vi "RT-PC Main.vi"() -> ()   [LabVIEW 2021]
panel:
  in  "[ESC]":bool
  in  "my name":string="name"
  in  "clear messages":bool
  in  "send datagrams":bool
  in  "listening port":u16=50001
  in  "destination port":u16=50001
  in  "destination IP":string
  out "my primary IP address":string
  out "my available IP addresses":string[](array[string])
  out "number of addresses":i32
  out "received datagrams":string
  # "UDP ping"
  # "restart VI after changing\nlistening port number"
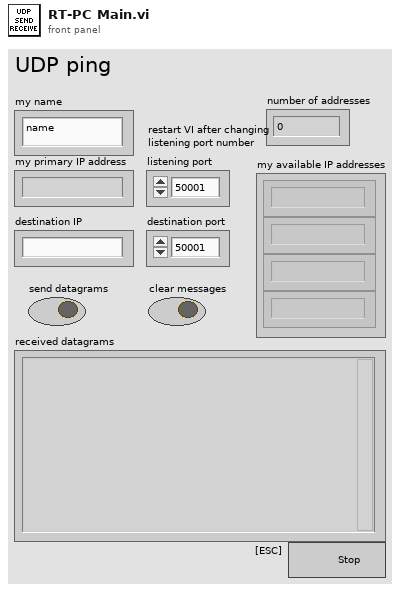
[diagram p1: front panel]
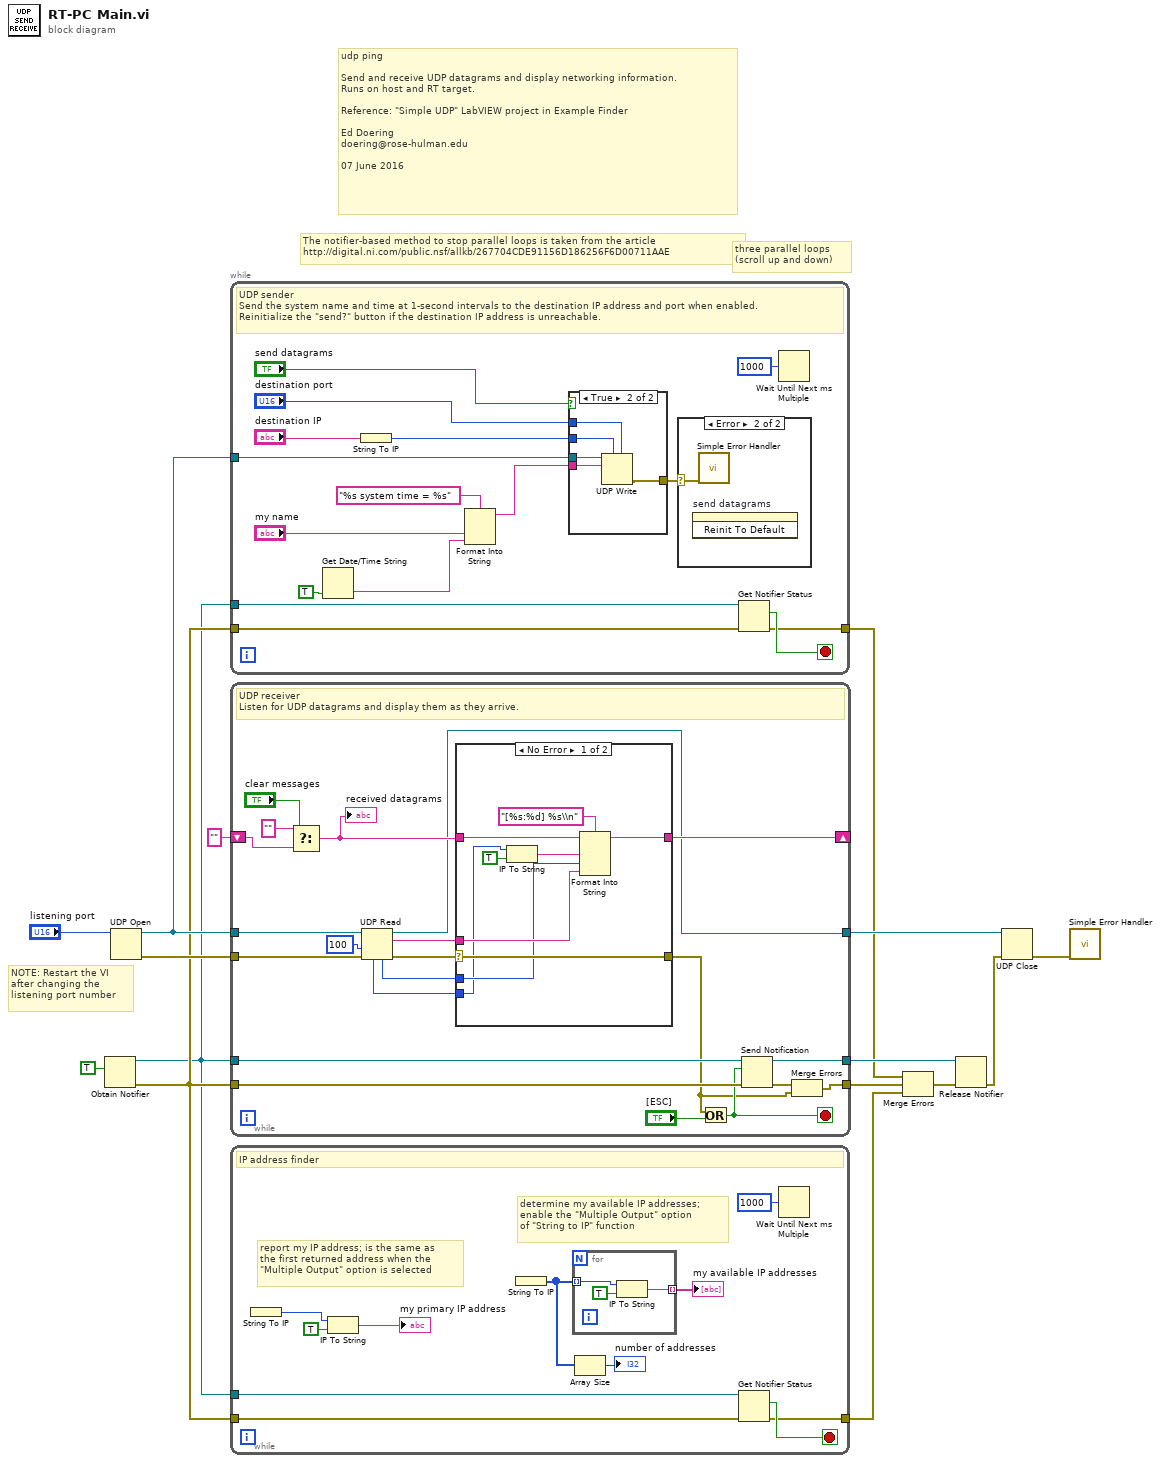
[diagram p0: block diagram]
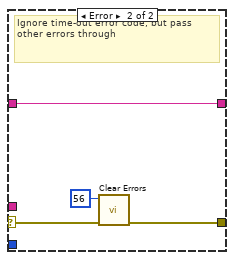
[diagram p4: hidden frame]
diagram:
  # "NOTE: Restart the VI\nafter changing the\nlistening port number"
  # "The notifier-based method to stop parallel loops is taken from the article\nhttp://digital.ni.com/public.nsf/allkb/267704CDE91156D186256F6D00711AAE"
  # "three parallel loops\n(scroll up and down)"
  # "udp ping\n\nSend and receive UDP datagrams and display networking information.\nRuns on host and RT target.\n\nReference: \"Simple UDP\" LabVIEW project in Example Finder \n\nEd Doering\ndoering@rose-hulman.edu\n\n07 June 2016"
  n1 = Obtain Notifier(notification data type=TRUE ("dot notation? (F)")) -> (notifier out=w2:refnum<notifier>, error out=w3:errorcluster)  [unwired: 3 in, 1 out]
  n2 = UDP Open(11:"listening port") -> (port=w12:refnum<k16>, 0:w14:errorcluster)  [unwired: 4 in, 1 out]
  n3 = while {
    tunnel: w12 -> [w27]
    tunnel: w3 -> [w19]
    tunnel: w2 -> [w18]
    tunnel: [w16] -> w1
    stop <- w17 stop-if-true
    # "UDP sender\nSend the system name and time at 1-second intervals to the destination IP address and port when enabled.\nReinitialize the \"send?\" button if the destination IP address is unreachable."
    n4 = Get Date/Time String(want seconds? (F)=TRUE) -> (time string=w26:string)  [unwired: 2 in, 1 out]
    n5 = String To IP(1:"destination IP") -> (0:w29:u32)
    n6 = Format Into String(format string="%s system time = %s", "my name", w26) -> (resulting string=w22:string)  [unwired: 2 in, 1 out]
    n7 = case shown="True" "send datagrams" {
      tunnel: w27 -> [_ w37]
      tunnel: [_ w36] -> w20
      tunnel: w22 -> [_ w35]
      tunnel: w29 -> [_ w34]
      tunnel: "destination port" -> [_ w33]
      frame False {
      }
      frame True {
        n8 = UDP Write(address=w34, port or service name=w33, connection ID=w37, data in=w35) -> (error out=w36:errorcluster)  [unwired: 2 in, 1 out]
      }
    }
    n9 = case shown="Error" w20 {
      selector: w20 -> [_ w32]
      frame No Error {
      }
      frame Error {
        n10 = invoke on="send datagrams" class="Bool (strict)" method="Reinit To Default"() -> ()  [unwired: 3 in, 3 out]
        n11 = call <vilib>:"Simple Error Handler.vi"("error in (no error)"=w32) -> ()  [unwired: 4 in, 5 out]
      }
    }
    n12 = Get Notifier Status(notifier=w18, error in (no error)=w19) -> (current notification=w17:bool, error out=w16:errorcluster)  [unwired: 3 out]
    n13 = Wait Until Next ms Multiple(millisecond multiple=u32 1000) -> ()  [unwired: 1 out]
  }
  n14 = while {
    tunnel: w12 -> [w58]
    tunnel: [w46] -> w15
    tunnel: w14 -> [w57]
    shift-right: [w55] -> _
    shift-left: "" -> [w50]
    tunnel: w2 -> [w45]
    tunnel: w3 -> [w44]
    tunnel: [w38] -> w4
    tunnel: [w41] -> w9
    stop <- w42 stop-if-true
    # "UDP receiver\nListen for UDP datagrams and display them as they arrive."
    n15 = Select(t="", s="clear messages", f=w50) -> (s? t:f=w47:string)
    "received datagrams" <- w47
    n16 = UDP Read(connection ID=w58, timeout ms (25000)=100, 8:w57) -> (data out=w54:string, error out=w56:errorcluster, 3:w46:refnum<k16>, 4:w53:u16, 6:w52:u32)  [unwired: 1 in]
    n17 = case shown="No Error" w56 {
      selector: w56 -> [w67 w70]
      tunnel: [w67 w69] -> w39
      tunnel: [w59 w71] -> w55
      tunnel: w47 -> [w60 w71]
      tunnel: w54 -> [w65 _]
      tunnel: w53 -> [w64 _]
      tunnel: w52 -> [w61 _]
      frame No Error {
        n18 = IP To String(1:TRUE ("dot notation? (F)"), 2:w61) -> (0:w62:string)
        n19 = Format Into String(format string="[%s:%d] %s\\n", initial string=w60, w62, w64, w65) -> (resulting string=w59:string)  [unwired: 1 in, 1 out]
      }
      frame Error {
        # "Ignore time-out error code, but pass other errors through"
        n20 = call <vilib>:"Clear Errors.vi"("error in (no error)"=w70, "specific error code to clear (0: all)"=56) -> ("error out"=w69:errorcluster)  [unwired: 4 in, 1 out]
      }
    }
    n21 = Or(x=w39, y="[ESC]") -> (x .or. y?=w42:bool)
    n22 = Send Notification(notification=w42, notifier=w45, error in (no error)=w44) -> (notifier out=w41:refnum<notifier>, error out=w40:errorcluster)
    n23 = Merge Errors(w40, w39) -> (w38:errorcluster)
  }
  n24 = while {
    tunnel: w3 -> [w75]
    tunnel: w2 -> [w74]
    tunnel: [w72] -> w8
    stop <- w73 stop-if-true
    # "determine my available IP addresses;\nenable the \"Multiple Output\" option\nof \"String to IP\" function"
    # "report my IP address; is the same as\nthe first returned address when the\n\"Multiple Output\" option is selected"
    # "IP address finder"
    n25 = String To IP() -> (0:w81:u32)  [unwired: 1 in]
    n26 = IP To String(1:TRUE ("dot notation? (F)"), 2:w81) -> (0:→"my primary IP address":string)
    n27 = String To IP() -> (0:w78:u32[])  [unwired: 1 in]
    n28 = for {
      tunnel: w78 -> [w84] mode=indexing
      tunnel: [w83] -> w79 mode=indexing
      n29 = IP To String(1:TRUE ("dot notation? (F)"), 2:w84) -> (0:w83:string)
    }
    "my available IP addresses" <- w79
    n30 = Array Size(array=w78) -> (size(s)=→"number of addresses":i32)
    n31 = Get Notifier Status(notifier=w74, error in (no error)=w75) -> (current notification=w73:bool, error out=w72:errorcluster)  [unwired: 3 out]
    n32 = Wait Until Next ms Multiple(millisecond multiple=u32 1000) -> ()  [unwired: 1 out]
  }
  n33 = Merge Errors(w1, w4, w8) -> (w7:errorcluster)
  n34 = Release Notifier(notifier=w9, error in (no error)=w7) -> (error out=w6:errorcluster)  [unwired: 1 in, 2 out]
  n35 = UDP Close(connection ID=w15, 8:w6) -> (error out=w5:errorcluster)  [unwired: 1 out]
  n36 = call <vilib>:"Simple Error Handler.vi"("error in (no error)"=w5) -> ()  [unwired: 4 in, 5 out]
